vi "Write Session Handle.vi"(8 "error in":errorcluster, 10 "Session Handle":T1, 11 "CPC in":refnum<class "CPC.lvclass">) -> (0 "error out":errorcluster, 3 "CPC out":refnum<class "CPC.lvclass">)   [LabVIEW 2014, in "CPC.lvclass"]
uses:
  CPC.lvclass
  reusable/Session APIs/Serial/Typedefs/Session Handle.ctl
  reusable/Session APIs/Serial/Serial Session.lvclass
  CPC.lvclass/CPC.ctl
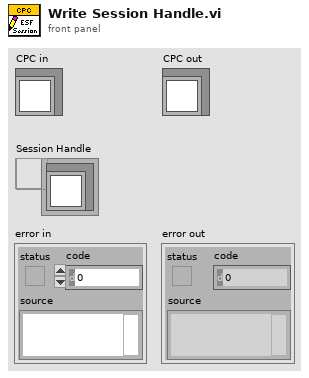
[diagram p1: front panel]
types:
  T1 = typedef "Serial Session.lvclass/Session Handle.ctl" = refnum<data-value>
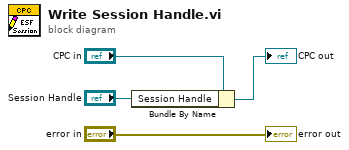
[diagram p0: block diagram]
diagram:
  n1 = Bundle By Name(cluster="CPC in", "Session Handle"="Session Handle") -> (→"CPC out":refnum<class "CPC.lvclass">)
  "error out" <- "error in"
